vi "subSave_AcquireTiCtrlInfomation.vi"(3 "TI-Ctrl":T1={"Obj"=6, "Cube Bottom"=1, "Cube Top"=4, "PFS-Ctrl"={"PFS IO"=FALSE, "PSF Err"=FALSE, "PSF Pos"=0}, "Z-Ctrl"={"Z-pos"=499.75, "Home"=TRUE, "Sensitivity"=1}, "Condenser"=2, "Lightpath"=enum."EYE"} {"Condenser" items=["A"=1, "DICN2"=2, "- empty 3 -"=3, "- empty 4 -"=4, "- empty 5 -"=5, "- empty 6 -"=6]; "Z-Ctrl"."Sensitivity" min=1 max=3 step=1 scale=1.0..3.0; "PFS-Ctrl"."PSF Pos" scale=0.0..16400.0; "Cube Top" items=["Cy5"=1, "TxRed"=2, "mO2"=3, "GFP-B"=4, "DAPI"=5, "- empty 6 -"=6]; "Cube Bottom" items=["- empty 1 -"=1, "- empty 2 -"=2, "- empty 3 -"=3, "- empty 4 -"=4, "- empty 5 -"=5, "- empty 6 -"=6]; "Obj" items=["20x/.75 Dry PFS"=1, " 40x/1.3 Oil PFS"=2, "60x/1.4 Oil PFS"=3, "- empty 4 -"=4, "- empty 5 -"=5, "- empty 6 -"=6]}) -> (1 "Text out":string)   [LabVIEW 2015]
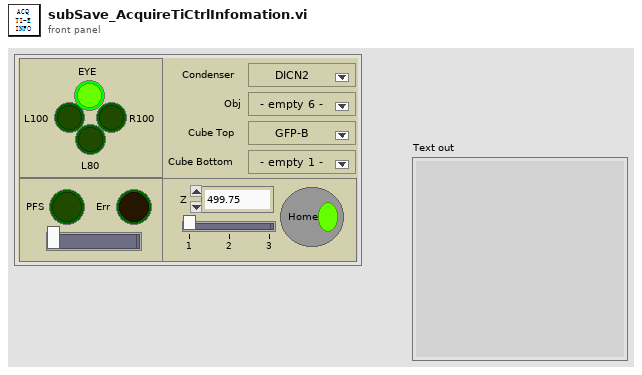
[diagram p1: front panel]
types:
  T1 = cluster{"Obj":u16, "Cube Bottom":u16, "Cube Top":u16, "PFS-Ctrl":cluster{"PFS IO":bool, "PSF Err":bool, "PSF Pos":u32}, "Z-Ctrl":cluster{"Z-pos":dbl, "Home":bool, "Sensitivity":u8}, "Condenser":u16, "Lightpath":enum32{"EYE", "L100", "R100", "L80"}}
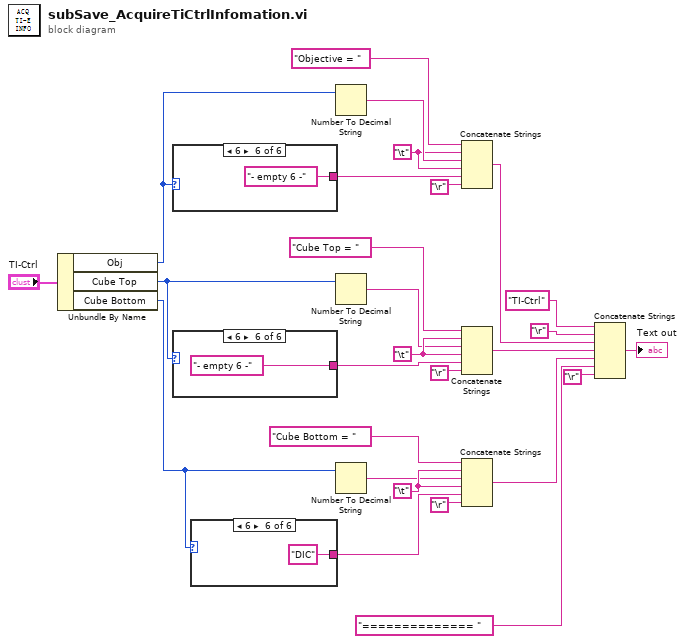
[diagram p0: block diagram]
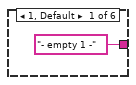
[diagram p2: hidden frame]
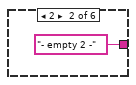
[diagram p3: hidden frame]
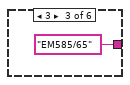
[diagram p4: hidden frame]
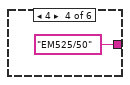
[diagram p5: hidden frame]
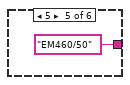
[diagram p6: hidden frame]
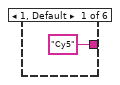
[diagram p7: hidden frame]
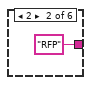
[diagram p8: hidden frame]
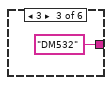
[diagram p9: hidden frame]
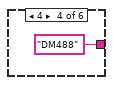
[diagram p10: hidden frame]
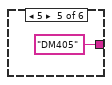
[diagram p11: hidden frame]
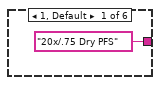
[diagram p12: hidden frame]
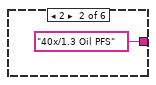
[diagram p13: hidden frame]
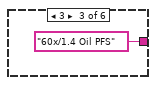
[diagram p14: hidden frame]
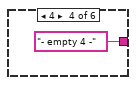
[diagram p15: hidden frame]
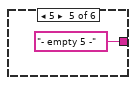
[diagram p16: hidden frame]
diagram:
  w18 = "\t"
  w12 = "\t"
  w1 = "\t"
  n1 = Unbundle By Name("TI-Ctrl") -> ("Obj"=w3:u16, "Cube Top"=w10:u16, "Cube Bottom"=w20:u16)
  n2 = case shown="6" w3 {
    tunnel: ["20x/.75 Dry PFS" ("string") "40x/1.3 Oil PFS" ("string") "60x/1.4 Oil PFS" ("string") "- empty 4 -" ("string") "- empty 5 -" ("string") "- empty 6 -" ("string")] -> w4
    frame 1, Default {
    }
    frame 2 {
    }
    frame 3 {
    }
    frame 4 {
    }
    frame 5 {
    }
    frame 6 {
    }
  }
  n3 = case shown="6" w10 {
    tunnel: ["Cy5" ("string") "RFP" ("string") "DM532" ("string") "DM488" ("string") "DM405" ("string") "- empty 6 -" ("string")] -> w13
    frame 1, Default {
    }
    frame 2 {
    }
    frame 3 {
    }
    frame 4 {
    }
    frame 5 {
    }
    frame 6 {
    }
  }
  n4 = case shown="6" w20 {
    tunnel: ["- empty 1 -" ("string") "- empty 2 -" ("string") "EM585/65" ("string") "EM525/50" ("string") "EM460/50" ("string") "DIC" ("string")] -> w19
    frame 1, Default {
    }
    frame 2 {
    }
    frame 3 {
    }
    frame 4 {
    }
    frame 5 {
    }
    frame 6 {
    }
  }
  n5 = Number To Decimal String(number=w3) -> (decimal integer string=w2:string)  [unwired: 1 in]
  n6 = Number To Decimal String(number=w10) -> (decimal integer string=w11:string)  [unwired: 1 in]
  n7 = Number To Decimal String(number=w20) -> (decimal integer string=w16:string)  [unwired: 1 in]
  n8 = Concatenate Strings("Objective = " ("string"), w1, w2, w1, w4, "\r") -> (w23:string)
  n9 = Concatenate Strings("Cube Top = " ("string"), w12, w11, w12, w13, "\r") -> (w24:string)
  n10 = Concatenate Strings("Cube Bottom = " ("string"), w18, w16, w18, w19, "\r") -> (w25:string)
  n11 = Concatenate Strings("TI-Ctrl" ("string"), "\r", w23, w24, w25, "============== " ("string"), "\r") -> (→"Text out":string)
